vi "CreateEvents.vi"(8 "error in (no error)":errorcluster, 11 "JQMHCore in":refnum<class "JQMHModule.lvclass">) -> (0 "error out":errorcluster, 3 "JQMHCore out":refnum<class "JQMHModule.lvclass">)   [LabVIEW 2024, in "JQMHModule.lvclass"]
uses:
  JQMHModule.lvclass
  StopEventArgs.ctl
  StandardEvents.ctl
  JQMHModule.lvclass/JQMHModule.ctl
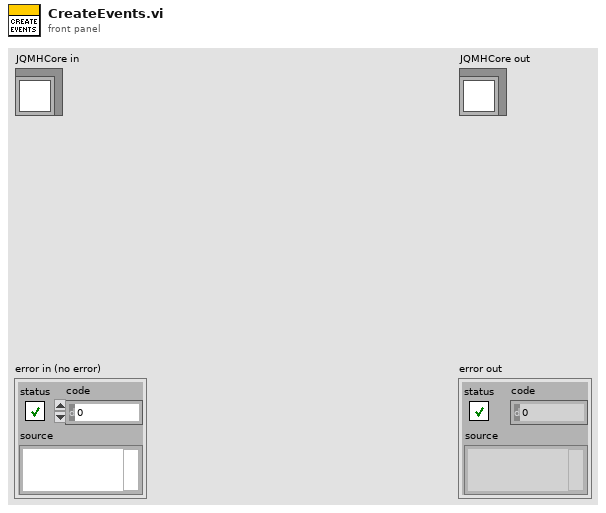
[diagram p1: front panel]
types:
  T1 = typedef "JQMHModule.lvclass/StandardEvents.ctl" = cluster{"Stop Module":refnum<user-event>}
  T2 = typedef "JQMHModule.lvclass/StopEventArgs.ctl" = bool
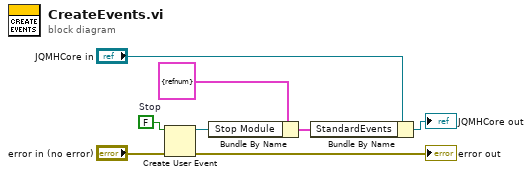
[diagram p0: block diagram]
diagram:
  w8 = T2 FALSE  # Stop
  n1 = Create User Event(user event datatype=w8, error in="error in (no error)") -> (user event=w2:refnum<user-event>, error out=→"error out":errorcluster)
  n2 = Bundle By Name(cluster=T1 {"Stop Module"=refnum} ("StandardEvents"), "Stop Module"=w2) -> (w1:T1)
  n3 = Bundle By Name(cluster="JQMHCore in", "StandardEvents"=w1) -> (→"JQMHCore out":refnum<class "JQMHModule.lvclass">)
